vi "create.path.vi"() -> (3 "Path":string)   [LabVIEW 2020, in "Run.lvclass"]
uses:
  Run.lvclass
  Run.lvclass/Run.ctl
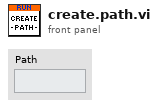
[diagram p1: front panel]
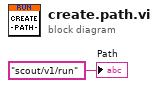
[diagram p0: block diagram]
diagram:
  "Path" <- "scout/v1/run"
